vi "蜂鸣器实验.vi"() -> ()   [LabVIEW 2011]
uses:
  <vilib>/eio/EIO_TerminalDirection.ctl
  <vilib>/STM32_DriverVI_Interface_F4/GPIO_EIO/GPO_EIO_Inner_F4.vi
  <vilib>/eio/EIONode/EIONode.xnode
panel:
  in  "毫秒倍数":u32(slide) scale=200.0..2000.0
  in  "停止":bool
  out "数值":i32
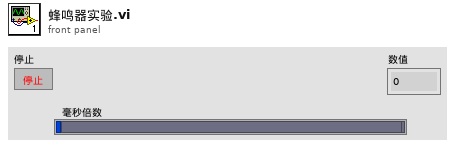
[diagram p1: front panel]
types:
  T1 = enum8{"P0", "P1", "P2", "P3", "P4", "P5", "P6", "P7", "P8", "P9", "P10", "P11", "P12", "P13", "P14", "P15"}
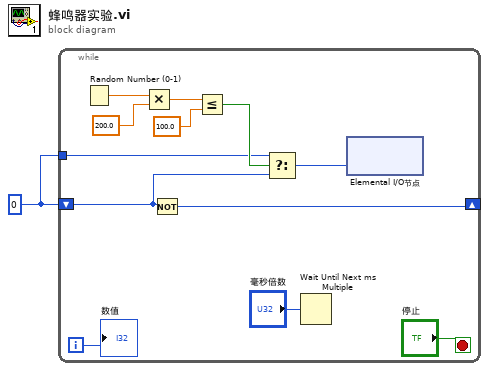
[diagram p0: block diagram]
diagram:
  w1 = u8 0 ("BEEP")
  n1 = while {
    shift-right: [w13] -> _
    shift-left: w1 -> [w3]
    tunnel: w1 -> [w2]
    i -> [w12]
    stop <- "停止" stop-if-true
    n2 = Random Number (0-1)() -> (number: 0 to 1=w9:dbl)
    n3 = Multiply(x=w9, y=200.0) -> (x*y=w7:dbl)
    n4 = Not(x=w3) -> (.not. x?=w13:u8)
    n5 = Less Or Equal?(x=w7, y=100.0) -> (x <= y?=w5:bool)
    n6 = Select(t=w2, s=w5, f=w3) -> (s? t:f=w4:u8)
    n7 = Wait Until Next ms Multiple(millisecond multiple="毫秒倍数") -> ()  [unwired: 1 out]
    n8 = xnode "Elemental I/O节点"("BEEP"=w4) -> ()  [unwired: 1 in, 1 out]
    "数值" <- w12
  }
